vi "Set DDS Loops Num.vi"(10 "num":cluster{}, 11 "channel_index":u8) -> ()   [LabVIEW 2021, in "vmmso.lvlib"]
doc: "DLL_API void WINAPI SetDDSLoopsNum(unsigned char channel_index, unsigned long long int num);"
uses:
  vmmso.lvlib
  vmmso.dll
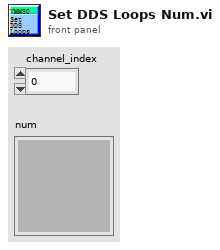
[diagram p1: front panel]
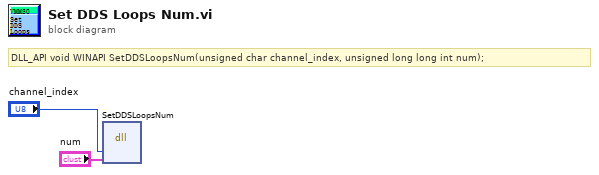
[diagram p0: block diagram]
diagram:
  # "DLL_API void WINAPI SetDDSLoopsNum(unsigned char channel_index, unsigned long long int num);"
  n1 = dll-call lib="D:/labviewdemo/LabviewDemo 21/vmmso/vmmso.*" fn="SetDDSLoopsNum"("channel_index"="channel_index", "num"="num") -> ()  [unwired: 6 in, 2 out]
